vi "DAC Init Results.vi"(8 "error in":errorcluster, 9 "Log Details?":bool, 10 "tdms file":refnum<k34>, 11 "DAC Shunt dU in":refnum<class "DAC Shunt dU.lvclass">) -> (0 "error out":errorcluster, 2 "tdms file out":refnum<k34>)   [LabVIEW 2019, in "DAC.lvlib" / "DAC Shunt dU.lvclass"]
uses:
  DAC Shunt dU.lvclass
  DAC.lvclass
  C:/Users/krio/Documents/LV_Projects/test-stand/App/DAC/DAC.lvclass
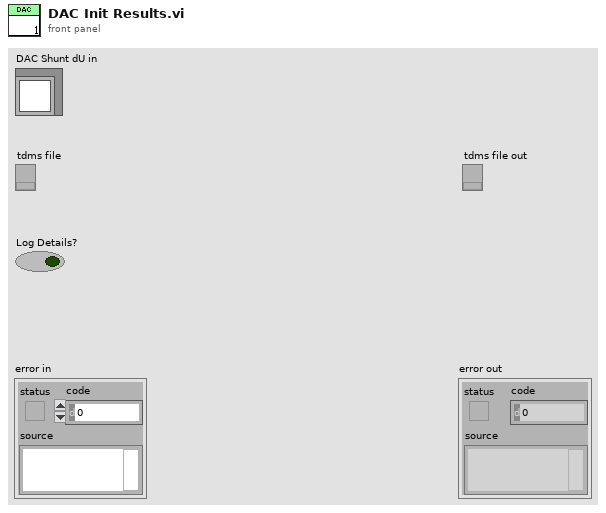
[diagram p1: front panel]
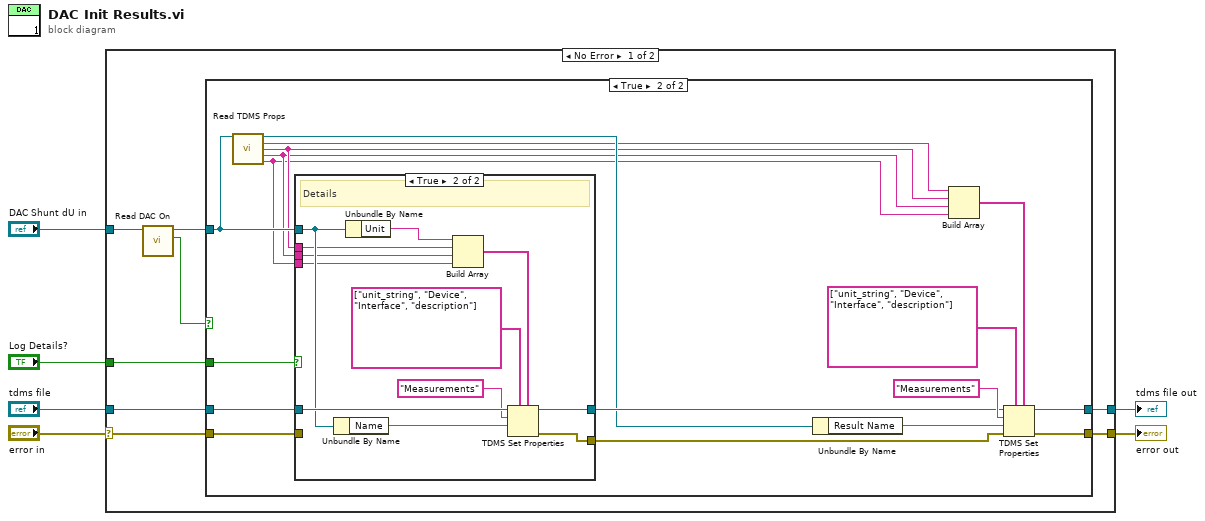
[diagram p0: block diagram]
diagram:
  n1 = case shown="No Error" "error in" {
    selector: "error in" -> [w8 w49]
    tunnel: [w12 w49] -> w6
    tunnel: "DAC Shunt dU in" -> [w11 _]
    tunnel: "tdms file" -> [w14 w48]
    tunnel: [w13 w48] -> w5
    tunnel: "Log Details?" -> [w7 _]
    frame No Error {
      n2 = call "Read DAC On.vi"("DAC in"=w11) -> ("DAC On"=w9:bool, "DAC out"=w10:refnum<class "DAC Shunt dU.lvclass">)  [unwired: 8 in, 1 out]
      n3 = case shown="True" w9 {
        tunnel: w14 -> [w15 w33]
        tunnel: [w15 w25] -> w13
        tunnel: [w16 w26] -> w12
        tunnel: w10 -> [_ w23]
        tunnel: w8 -> [w16 w24]
        tunnel: w7 -> [_ w32]
        frame False {
        }
        frame True {
          n4 = call "Read TDMS Props.vi"("DAC in"=w23) -> ("DAC out"=w22:refnum<class "DAC Shunt dU.lvclass">, "Result Unit"=w20:string, "DAC Device"=w19:string, "DAC IO"=w18:string, "DAC Description"=w17:string)  [unwired: 10 in]
          n5 = case shown="True" w32 {
            tunnel: w33 -> [w35 w47]
            tunnel: [w35 w43] -> w28
            tunnel: [w34 w42] -> w27
            tunnel: w23 -> [_ w40]
            tunnel: w24 -> [w34 _]
            tunnel: w19 -> [_ w38]
            tunnel: w18 -> [_ w37]
            tunnel: w17 -> [_ w36]
            frame False {
            }
            frame True {
              # "Details"
              n6 = Unbundle By Name(w40) -> ("Name"=w41:string)
              n7 = Unbundle By Name(w40) -> ("Unit"=w45:string)
              n8 = Build Array(w45, w38, w37, w36) -> (w44:string[])
              n9 = TDMS Set Properties(5:w44, 7:string[] ["unit_string", "Device", "Interface", "description"] ("property names"), 9:w41, 10:"Measurements" ("group name in (Untitled)"), 11:w47) -> (0:w42:errorcluster, 3:w43:refnum<k34>)  [unwired: 1 in, 2 out]
            }
          }
          n10 = Unbundle By Name(w22) -> ("Result Name"=w29:string)
          n11 = Build Array(w20, w19, w18, w17) -> (w30:string[])
          n12 = TDMS Set Properties(5:w30, 7:string[] ["unit_string", "Device", "Interface", "description"] ("property names"), 8:w27, 9:w29, 10:"Measurements" ("group name in (Untitled)"), 11:w28) -> (0:w26:errorcluster, 3:w25:refnum<k34>)  [unwired: 2 out]
        }
      }
    }
    frame Error {
    }
  }
  "error out" <- w6
  "tdms file out" <- w5
